vi "MIDI-Parser.vi"(8 "Error In":errorcluster, 11 "Consumer Data In":T3={"Queue_Consumer"=refnum, "Selected Consumer"=enum."Random", "Session Data"={"Tx-Data"=[], "Rx-Data"=[], "MIDI-Message log"=[{"Message Name"="", "Meta value"=0, "Datastring"="", "Datatype"=enum."No Data"}]}, "Timout-Time[ms]"=0, "To_GUI-Consumer"=refnum, "CPU(ms)"=0, "Console log"="", "MIDI Parse Data"={"MIDI-Bytes In"=[145, 60, 100], "MIDI Tag"=[], "MIDI Parsed Data"=[], "Iteration"=0, "Error?"=[], "Running States"=[], "Running Statusbyte"=0, "Running StatusString"="", "Third Byte Flag"=FALSE, "Current Byte"=0, "Sysex"="", "Expect Databyte"=FALSE}, "Session Inspection Data"={"Diff"=[], "Tx Byte"=[], "Rx Byte"=[], "Send Log"=[], "Parsed Data"={"Tx MIDI Tag"=[], "Tx MIDI Parsed Data"=[], "Tx Error"=[], "Tx Running States"=[], "Rx MIDI Tag"=[], "Rx MIDI Parsed Data"=[], "Rx Error"=[], "Rx Running States"=[], "Diff"=[]}}} {"MIDI Parse Data"."Current Byte" format="%.0x"; "MIDI Parse Data"."Running Statusbyte" format="%.0x"; "MIDI Parse Data"."MIDI-Bytes In" format="%.0x"}) -> (0 "Error Out":errorcluster, 3 "Consumer Data Out":T3={"Queue_Consumer"=refnum, "Selected Consumer"=enum."Random", "Session Data"={"Tx-Data"=[], "Rx-Data"=[], "MIDI-Message log"=[{"Message Name"="", "Meta value"=0, "Datastring"="", "Datatype"=enum."No Data"}]}, "Timout-Time[ms]"=0, "To_GUI-Consumer"=refnum, "CPU(ms)"=0, "Console log"="", "MIDI Parse Data"={"MIDI-Bytes In"=[145, 60, 100], "MIDI Tag"=[], "MIDI Parsed Data"=[], "Iteration"=0, "Error?"=[], "Running States"=[], "Running Statusbyte"=0, "Running StatusString"="", "Third Byte Flag"=FALSE, "Current Byte"=0, "Sysex"="", "Expect Databyte"=FALSE}, "Session Inspection Data"={"Diff"=[], "Tx Byte"=[], "Rx Byte"=[], "Send Log"=[], "Parsed Data"={"Tx MIDI Tag"=[], "Tx MIDI Parsed Data"=[], "Tx Error"=[], "Tx Running States"=[], "Rx MIDI Tag"=[], "Rx MIDI Parsed Data"=[], "Rx Error"=[], "Rx Running States"=[], "Diff"=[]}}} {"MIDI Parse Data"."Current Byte" format="%.0x"; "MIDI Parse Data"."Running Statusbyte" format="%.0x"; "MIDI Parse Data"."MIDI-Bytes In" format="%.0x"})   [LabVIEW 2019]
doc: "This parser constructs MIDI-messages from bytearray, by following the MIDI-spec."
uses:
  Controls/Parser-data.ctl
  Controls/Consumer_Data.ctl
  Common/Controls/Application_Message.ctl
  Common/Controls/Application_State.ctl
  Controls/Consumer_States.ctl
  Controls/Transfer_Data.ctl
  MIDI/Controls/MIDI-Message_Array.ctl
  MIDI/Controls/MIDI-Message_Cluster.ctl
  MIDI/Controls/Meta_Commands.ctl
  Controls/Consumer_Result.ctl
  Controls/Parsed_Data.ctl
  Controls/MIDI-States.ctl
panel:
  out "Control Tab":T1(tab)
  out "Console Out":string
  in  "MIDI Parse Data":T2={"MIDI-Bytes In"=[145, 60, 100], "MIDI Tag"=[], "MIDI Parsed Data"=[], "Iteration"=0, "Error?"=[], "Running States"=[], "Running Statusbyte"=0, "Running StatusString"="", "Third Byte Flag"=FALSE, "Current Byte"=0, "Sysex"="", "Expect Databyte"=FALSE} {"Current Byte" format="%.0x"; "Running Statusbyte" format="%.0x"; "MIDI-Bytes In" format="%.0x"}
  out "MIDI Tag":string[](array[string])
  out "MIDI Parsed Data":string[](array[string])
  out "Running States":string[](array[string])
  out "Error?":bool[](array[boolean])
  out "Error Message":string
  out "VI-filename":string
  out "Revision Number":u32
  out "VI Description":string
  out "Callers' Names":string[](array[string])
  out "Code Size":u32
  out "VI Type":T11(ring)
  out "Project name":string
  out "Project filepath":path
  out "VI filepath":path
  out "Project Description":string
  out "VI-Name":string
  in  "Stop":bool
  # "Common Errors:"
  # "0:"
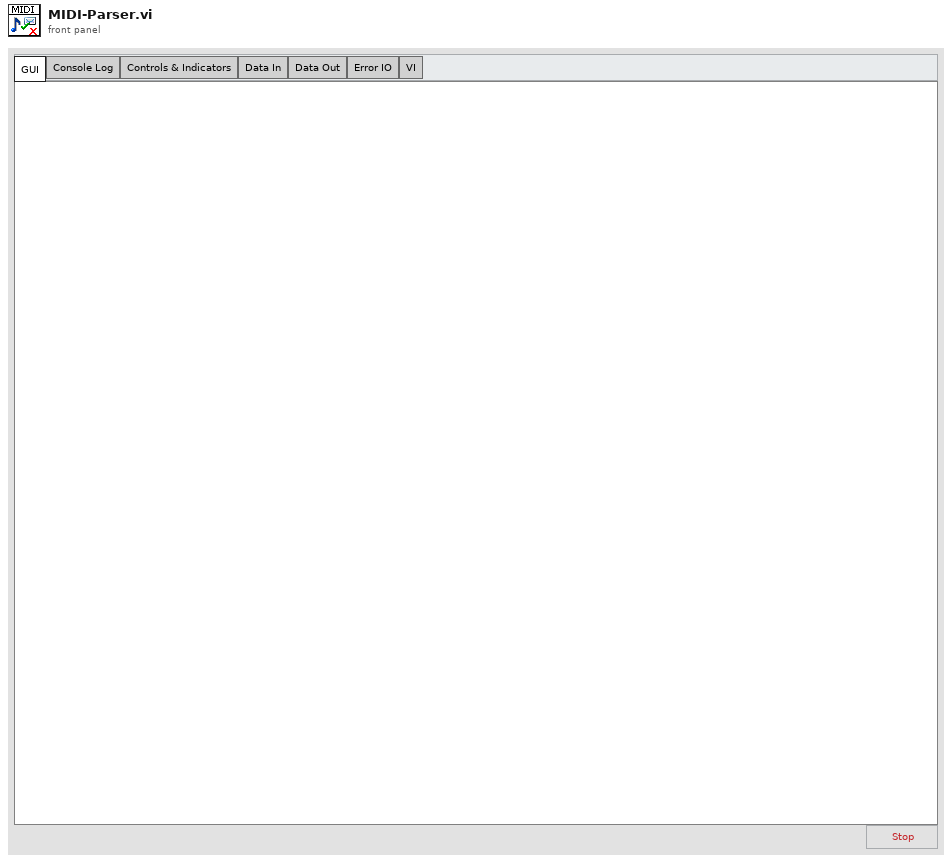
[diagram p1: front panel]
types:
  T1 = enum32{"GUI", "Console Log", "Controls & Indicators", "Data In", "Data Out", "Error IO", "VI"}
  T2 = typedef "Parser-data.ctl" = cluster{"MIDI-Bytes In":u8[], "MIDI Tag":string[], "MIDI Parsed Data":string[], "Iteration":i32, "Error?":bool[], "Running States":string[], "Running Statusbyte":u8, "Running StatusString":string, "Third Byte Flag":bool, "Current Byte":u8, "Sysex":string, "Expect Databyte":bool}
  T3 = typedef "Consumer_Data.ctl" = cluster{"Queue_Consumer":refnum<queue>, "Selected Consumer":T4, "Session Data":T5, "Timout-Time[ms]":i32, "To_GUI-Consumer":refnum<user-event>, "CPU(ms)":u32, "Console log":string, "MIDI Parse Data":T2, "Session Inspection Data":T9}
  T4 = typedef "Consumer_States.ctl" = enum16{"Random", "ECG", "Strech-Patch"}
  T5 = typedef "Transfer_Data.ctl" = cluster{"Tx-Data":i8[], "Rx-Data":i8[], "MIDI-Message log":T6}
  T6 = typedef "MIDI-Message_Array.ctl" = T7[]
  T7 = typedef "MIDI-Message_Cluster.ctl" = cluster{"Message Name":string, "Meta value":i32, "Datastring":string, "Datatype":T8}
  T8 = typedef "Meta_Commands.ctl" = enum16{"No Data", "Pause", "Loop", "Wait for Rx", "Delay", "Break", "MIDI"}
  T9 = typedef "Consumer_Result.ctl" = cluster{"Diff":bool[], "Tx Byte":string[], "Rx Byte":string[], "Send Log":string[], "Parsed Data":T10}
  T10 = typedef "Parsed_Data.ctl" = cluster{"Tx MIDI Tag":string[], "Tx MIDI Parsed Data":string[], "Tx Error":bool[], "Tx Running States":string[], "Rx MIDI Tag":string[], "Rx MIDI Parsed Data":string[], "Rx Error":bool[], "Rx Running States":string[], "Diff":bool[]}
  T11 = enum32{"invalid VI type", "Standard VI", "Control VI", "Global VI", "Polymorphic VI", "Configuration VI", "SubSystem", "Facade VI", "Method VI", "Statechart Diagram VI"}
  T12 = typedef "MIDI-States.ctl" = enum16{"Init Reset", "Dispatch Status", "SysEx"}
  T13 = typedef "LVRectTypeDef.ctl" = cluster{"Left":i16, "Top":i16, "Right":i16, "Bottom":i16}
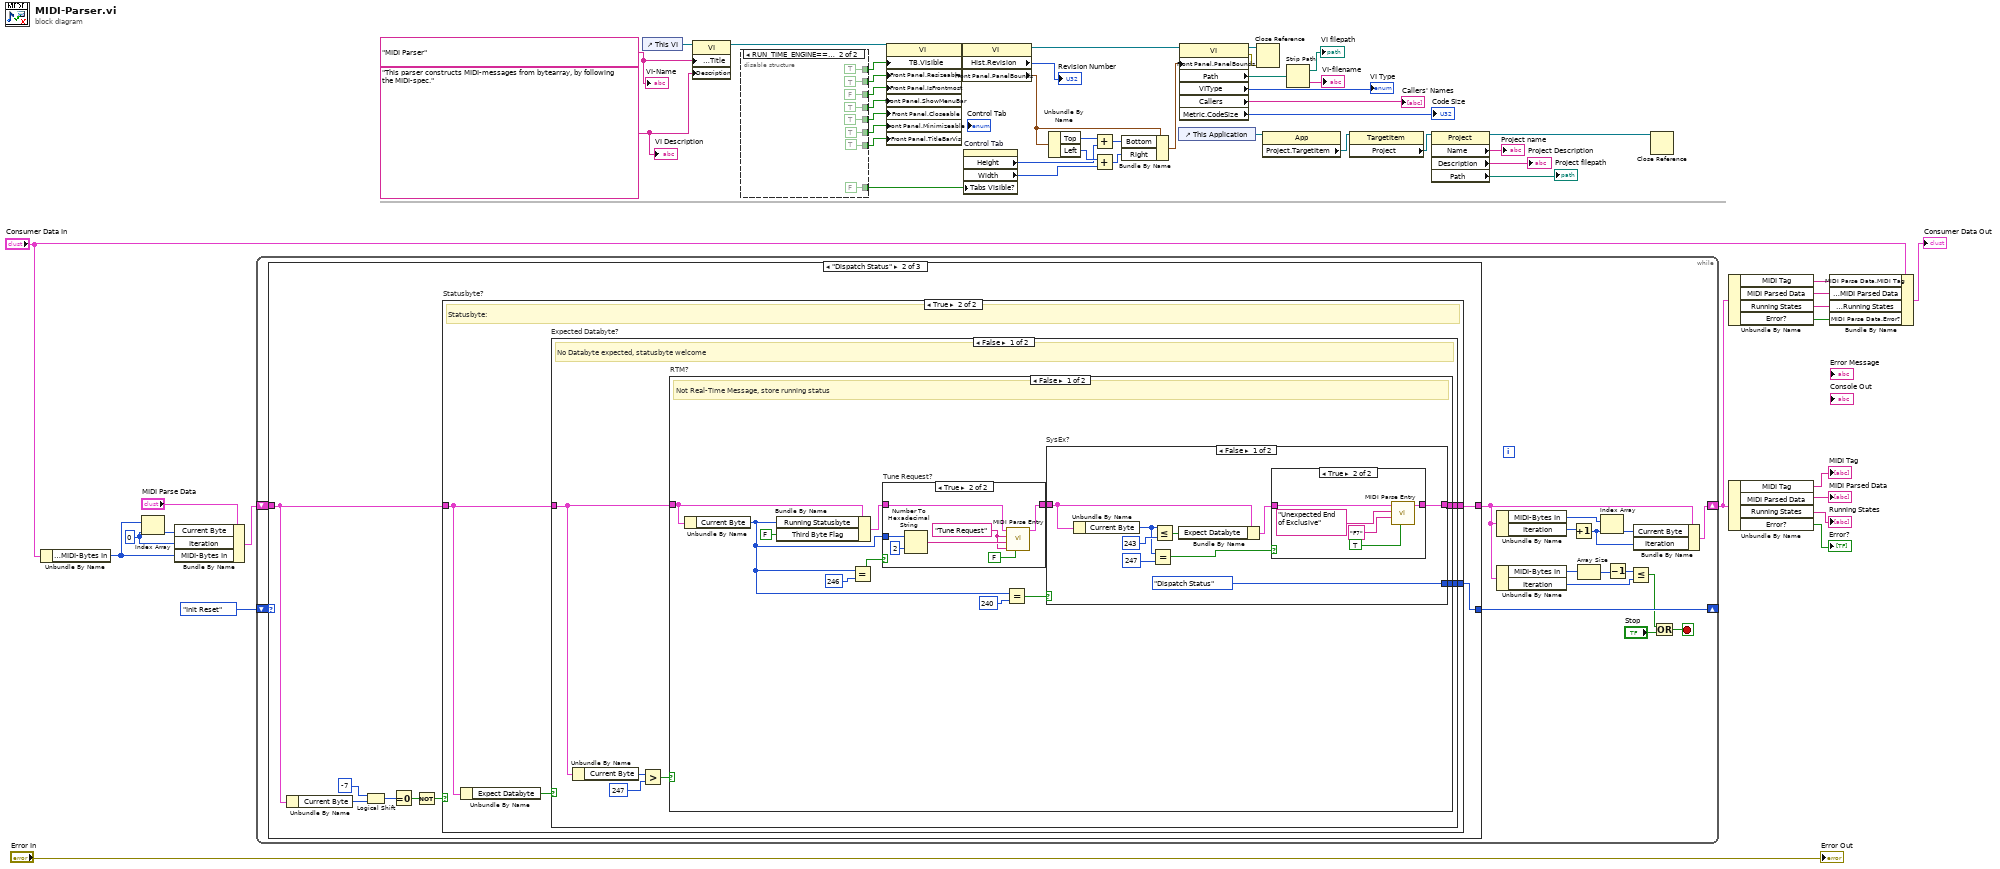
[diagram p0: block diagram]
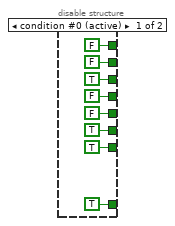
[diagram p2: hidden frame]
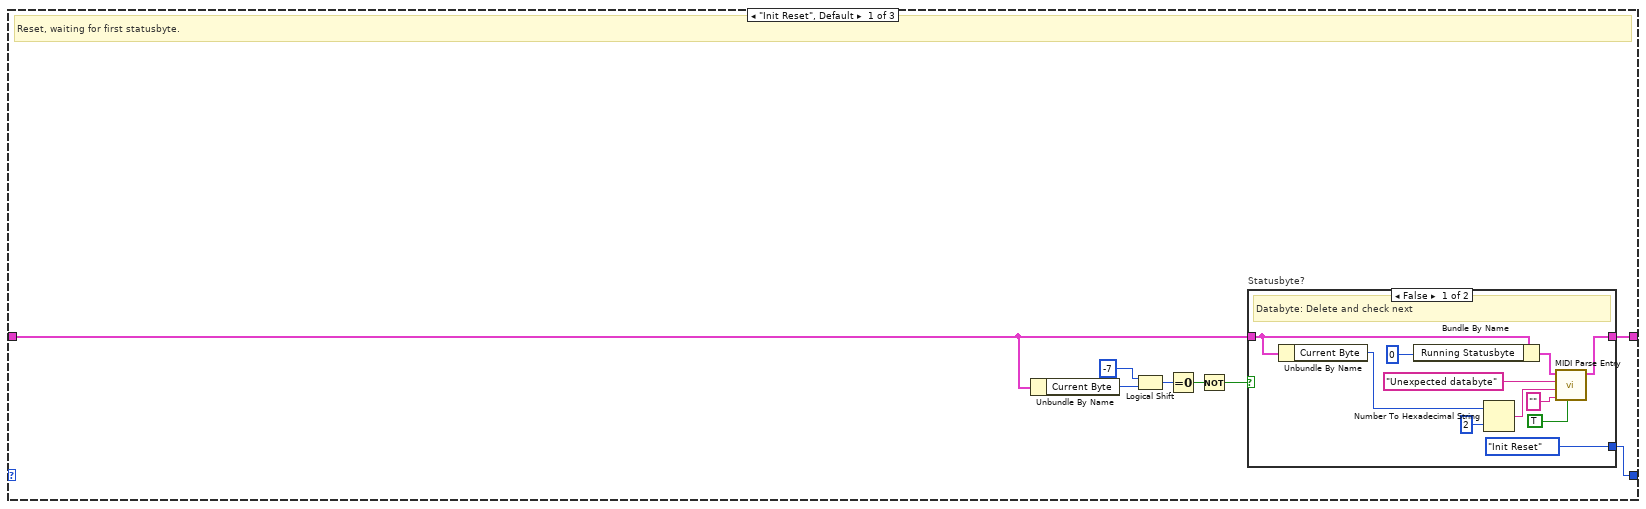
[diagram p3: hidden frame]
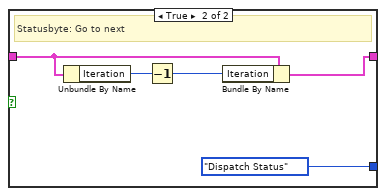
[diagram p4: hidden frame]
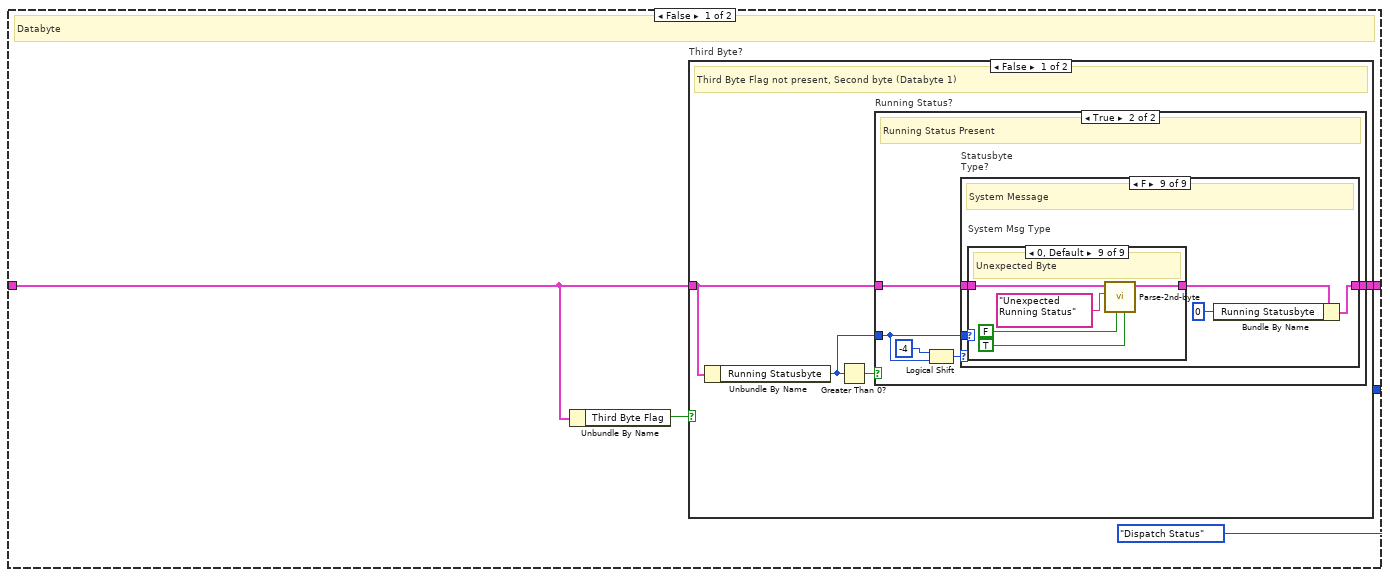
[diagram p5: hidden frame]
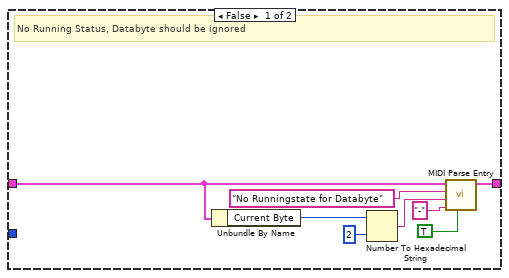
[diagram p6: hidden frame]
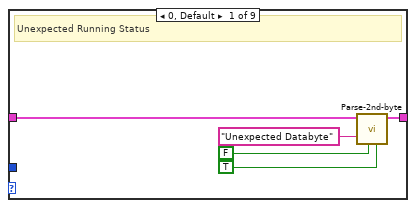
[diagram p7: hidden frame]
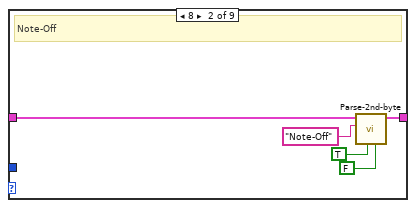
[diagram p8: hidden frame]
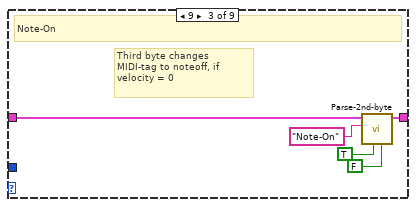
[diagram p9: hidden frame]
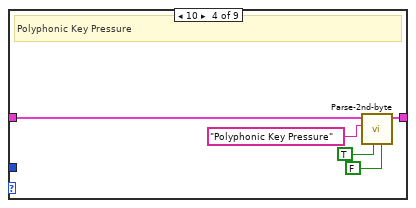
[diagram p10: hidden frame]
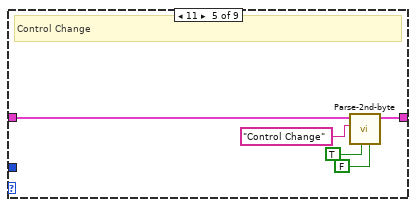
[diagram p11: hidden frame]
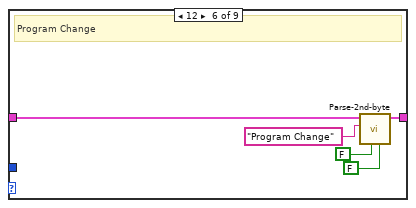
[diagram p12: hidden frame]
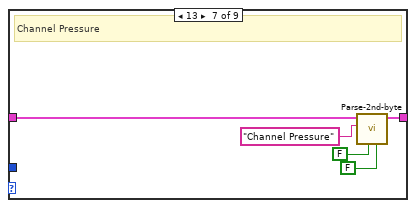
[diagram p13: hidden frame]
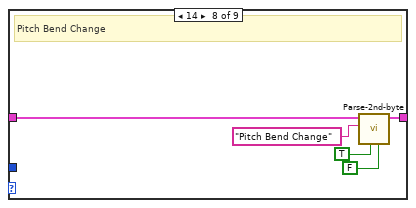
[diagram p14: hidden frame]
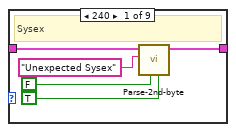
[diagram p15: hidden frame]
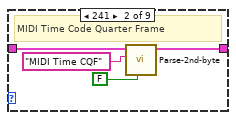
[diagram p16: hidden frame]
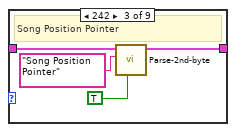
[diagram p17: hidden frame]
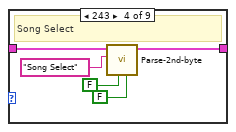
[diagram p18: hidden frame]
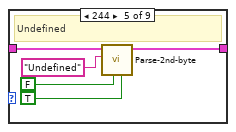
[diagram p19: hidden frame]
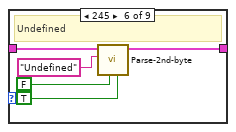
[diagram p20: hidden frame]
diagram:
  w42 = "MIDI Parser"
  w41 = "This parser constructs MIDI-messages from bytearray, by following the MIDI-spec."
  w52 = 0
  n1 = Unbundle By Name("Consumer Data In") -> ("MIDI Parse Data.MIDI-Bytes In"=w11:u8[])
  n2 = Index Array(array=w11, index=w52) -> (element=w51:u8)
  n3 = Bundle By Name(cluster="MIDI Parse Data", "Current Byte"=w51, "Iteration"=w52, "MIDI-Bytes In"=w11) -> (w56:T2)
  n4 = while {
    shift-right: [w67] -> w1
    shift-left: w56 -> [w72]
    shift-right: [w71] -> _
    shift-left: MIDI-States."Init Reset" -> [w73]
    stop <- w61 stop-if-true
    n5 = case shown="\"Dispatch Status\"" w73 {
      tunnel: w72 -> [w79 w101 w358]
      tunnel: [w78 w98 w355] -> w71
      tunnel: [w81 w100 w356] -> w65
      frame "Init Reset", Default {
        # "Reset, waiting for first statusbyte."
        n6 = Unbundle By Name(w79) -> ("Current Byte"=w80:u8)
        n7 = Logical Shift(y=i16 -7, x=w80) -> (x << y=w76:u8)
        n8 = Equal To 0?(x=w76) -> (x = 0?=w75:bool)
        n9 = Not(x=w75) -> (.not. x?=w74:bool)
        n10 = case "Statusbyte?" shown="False" w74 {
          tunnel: w79 -> [w86 w94]
          tunnel: [w84 w93] -> w81
          tunnel: [MIDI-States."Init Reset" MIDI-States."Dispatch Status"] -> w78
          frame False {
            # "Databyte: Delete and check next"
            n11 = Unbundle By Name(w86) -> ("Current Byte"=w82:u8)
            n12 = Bundle By Name(cluster=w86, "Running Statusbyte"=u8 0 ("Running Status")) -> (w85:T2)
            n13 = Number To Hexadecimal String(1:i16 2 ("width (-)"), 2:w82) -> (0:w87:string)
            n14 = call "MIDI Parse Entry.vi"("Error"=TRUE, "Running State"="", "Datastring"=w87, "MIDI Tag"="Unexpected databyte", "MIDI Parse Data in"=w85) -> ("MIDI Parse Data out"=w84:T2)  [unwired: 6 in]
          }
          frame True {
            # "Statusbyte: Go to next"
            n15 = Unbundle By Name(w94) -> ("Iteration"=w96:i32)
            n16 = Decrement(x=w96) -> (x-1=w95:i32)
            n17 = Bundle By Name(cluster=w94, "Iteration"=w95) -> (w93:T2)
          }
        }
      }
      frame "Dispatch Status" {
        n18 = Unbundle By Name(w101) -> ("Current Byte"=w99:u8)
        n19 = Logical Shift(y=i16 -7, x=w99) -> (x << y=w104:u8)
        n20 = Equal To 0?(x=w104) -> (x = 0?=w103:bool)
        n21 = Not(x=w103) -> (.not. x?=w102:bool)
        n22 = case "Statusbyte?" shown="True" w102 {
          tunnel: w101 -> [w108 w243]
          tunnel: [w107 w245] -> w100
          tunnel: [MIDI-States."Dispatch Status" w244] -> w98
          frame False {
            # "Databyte"
            n23 = Unbundle By Name(w108) -> ("Third Byte Flag"=w109:bool)
            n24 = case "Third Byte?" shown="False" w109 {
              tunnel: w108 -> [w112 w233]
              tunnel: [w110 w221] -> w107
              frame False {
                # "Third Byte Flag not present, Second byte (Databyte 1)"
                n25 = Unbundle By Name(w112) -> ("Running Statusbyte"=w111:u8)
                n26 = Greater Than 0?(x=w111) -> (x > 0?=w113:bool)
                n27 = case "Running Status?" shown="True" w113 {
                  tunnel: w112 -> [w115 w124]
                  tunnel: w111 -> [_ w123]
                  tunnel: [w114 w122] -> w110
                  frame False {
                    # "No Running Status, Databyte should be ignored"
                    n28 = Unbundle By Name(w115) -> ("Current Byte"=w116:u8)
                    n29 = Number To Hexadecimal String(1:i16 2 ("width (-)"), 2:w116) -> (0:w117:string)
                    n30 = call "MIDI Parse Entry.vi"("Error"=TRUE, "Running State"="-", "Datastring"=w117, "MIDI Tag"="No Runningstate for Databyte", "MIDI Parse Data in"=w115) -> ("MIDI Parse Data out"=w114:T2)  [unwired: 6 in]
                  }
                  frame True {
                    # "Running Status Present"
                    n31 = Logical Shift(y=i16 -4, x=w123) -> (x << y=w125:u8)
                    n32 = case "Statusbyte\nType?" shown="F" w125 {
                      tunnel: w124 -> [w129 w135 w140 w145 w150 w155 w160 w165 w170]
                      tunnel: w123 -> [_ _ _ _ _ _ _ _ w171]
                      tunnel: [w127 w134 w139 w146 w149 w154 w159 w164 w168] -> w122
                      frame 0, Default {
                        # "Unexpected Running Status"
                        n33 = call "Parse-2nd-byte.vi"("Error?"=TRUE, "Third Byte Flag"=FALSE, "Statustype"="Unexpected Databyte", "MIDI Parse Data in"=w129) -> ("MIDI Parse Data out"=w127:T2)  [unwired: 7 in]
                      }
                      frame 8 {
                        # "Note-Off"
                        n34 = call "Parse-2nd-byte.vi"("Error?"=FALSE, "Third Byte Flag"=TRUE, "Statustype"="Note-Off", "MIDI Parse Data in"=w135) -> ("MIDI Parse Data out"=w134:T2)  [unwired: 7 in]
                      }
                      frame 9 {
                        # "Third byte changes MIDI-tag to noteoff, if velocity = 0"
                        # "Note-On"
                        n35 = call "Parse-2nd-byte.vi"("Error?"=FALSE, "Third Byte Flag"=TRUE, "Statustype"="Note-On", "MIDI Parse Data in"=w140) -> ("MIDI Parse Data out"=w139:T2)  [unwired: 7 in]
                      }
                      frame 10 {
                        # "Polyphonic Key Pressure"
                        n36 = call "Parse-2nd-byte.vi"("Error?"=FALSE, "Third Byte Flag"=TRUE, "Statustype"="Polyphonic Key Pressure", "MIDI Parse Data in"=w145) -> ("MIDI Parse Data out"=w146:T2)  [unwired: 7 in]
                      }
                      frame 11 {
                        # "Control Change"
                        n37 = call "Parse-2nd-byte.vi"("Error?"=FALSE, "Third Byte Flag"=TRUE, "Statustype"="Control Change", "MIDI Parse Data in"=w150) -> ("MIDI Parse Data out"=w149:T2)  [unwired: 7 in]
                      }
                      frame 12 {
                        # "Program Change"
                        n38 = call "Parse-2nd-byte.vi"("Error?"=FALSE, "Third Byte Flag"=FALSE, "Statustype"="Program Change", "MIDI Parse Data in"=w155) -> ("MIDI Parse Data out"=w154:T2)  [unwired: 7 in]
                      }
                      frame 13 {
                        # "Channel Pressure"
                        n39 = call "Parse-2nd-byte.vi"("Error?"=FALSE, "Third Byte Flag"=FALSE, "Statustype"="Channel Pressure", "MIDI Parse Data in"=w160) -> ("MIDI Parse Data out"=w159:T2)  [unwired: 7 in]
                      }
                      frame 14 {
                        # "Pitch Bend Change"
                        n40 = call "Parse-2nd-byte.vi"("Error?"=FALSE, "Third Byte Flag"=TRUE, "Statustype"="Pitch Bend Change", "MIDI Parse Data in"=w165) -> ("MIDI Parse Data out"=w164:T2)  [unwired: 7 in]
                      }
                      frame 15 {
                        # "System Message"
                        n41 = case "System Msg Type" shown="0, Default" w171 {
                          tunnel: w170 -> [w174 w179 w182 w187 w191 w196 w202 w206 w211]
                          tunnel: [w173 w178 w181 w186 w190 w195 w201 w205 w210] -> w169
                          frame 240 {
                            # "Sysex"
                            n42 = call "Parse-2nd-byte.vi"("Error?"=TRUE, "Third Byte Flag"=FALSE, "Statustype"="Unexpected Sysex", "MIDI Parse Data in"=w174) -> ("MIDI Parse Data out"=w173:T2)  [unwired: 7 in]
                          }
                          frame 241 {
                            # "MIDI Time Code Quarter Frame"
                            n43 = call "Parse-2nd-byte.vi"("Third Byte Flag"=FALSE, "Statustype"="MIDI Time CQF", "MIDI Parse Data in"=w179) -> ("MIDI Parse Data out"=w178:T2)  [unwired: 8 in]
                          }
                          frame 242 {
                            # "Song Position Pointer"
                            n44 = call "Parse-2nd-byte.vi"("Third Byte Flag"=TRUE, "Statustype"="Song Position Pointer", "MIDI Parse Data in"=w182) -> ("MIDI Parse Data out"=w181:T2)  [unwired: 8 in]
                          }
                          frame 243 {
                            # "Song Select"
                            n45 = call "Parse-2nd-byte.vi"("Error?"=FALSE, "Third Byte Flag"=FALSE, "Statustype"="Song Select", "MIDI Parse Data in"=w187) -> ("MIDI Parse Data out"=w186:T2)  [unwired: 7 in]
                          }
                          frame 244 {
                            # "Undefined"
                            n46 = call "Parse-2nd-byte.vi"("Error?"=TRUE, "Third Byte Flag"=FALSE, "Statustype"="Undefined", "MIDI Parse Data in"=w191) -> ("MIDI Parse Data out"=w190:T2)  [unwired: 7 in]
                          }
                          frame 245 {
                            # "Undefined"
                            n47 = call "Parse-2nd-byte.vi"("Error?"=TRUE, "Third Byte Flag"=FALSE, "Statustype"="Undefined", "MIDI Parse Data in"=w196) -> ("MIDI Parse Data out"=w195:T2)  [unwired: 7 in]
                          }
                          frame 246 {
                            # "Tune Request"
                            n48 = call "Parse-2nd-byte.vi"("Error?"=TRUE, "Third Byte Flag"=FALSE, "Statustype"="Unexpected TQ", "MIDI Parse Data in"=w202) -> ("MIDI Parse Data out"=w201:T2)  [unwired: 7 in]
                          }
                          frame 247 {
                            # "End of Exclusive"
                            n49 = call "Parse-2nd-byte.vi"("Error?"=TRUE, "Third Byte Flag"=FALSE, "Statustype"="Unexpected End of Exclusive", "MIDI Parse Data in"=w206) -> ("MIDI Parse Data out"=w205:T2)  [unwired: 7 in]
                          }
                          frame 0, Default {
                            # "Unexpected Byte"
                            n50 = call "Parse-2nd-byte.vi"("Error?"=TRUE, "Third Byte Flag"=FALSE, "Statustype"="Unexpected Running Status", "MIDI Parse Data in"=w211) -> ("MIDI Parse Data out"=w210:T2)  [unwired: 7 in]
                          }
                        }
                        n51 = Bundle By Name(cluster=w169, "Running Statusbyte"=u8 0) -> (w168:T2)
                      }
                    }
                  }
                }
              }
              frame True {
                w215 = FALSE ("Third Byte Flag")
                # "Designate as Note off, if velocity is 0 on Note-on"
                # "Third byte"
                n52 = Unbundle By Name(w233) -> ("MIDI Parsed Data"=w235:string[], "Current Byte"=w216:u8, "MIDI Tag"=w225:string[], "Running Statusbyte"=w228:u8)
                n53 = Array Size(array=w235) -> (size(s)=w239:i32)
                n54 = Decrement(x=w239) -> (x-1=w238:i32)
                n55 = Logical Shift(y=i16 -4, x=w228) -> (x << y=w230:u8)
                n56 = Index Array(array=w235, index=w238) -> (element=w237:string)
                n57 = Number To Hexadecimal String(1:i16 2 ("width (-)"), 2:w216) -> (0:w240:string)
                n58 = Array Size(array=w225) -> (size(s)=w227:i32)
                n59 = Decrement(x=w227) -> (x-1=w226:i32)
                n60 = Array Size(array=w235) -> (size(s)=w234:i32)
                n61 = Replace Array Subset(array=w225, new element="Note-Off*" ("new element/subarray"), index=w226) -> (w224:string[])
                n62 = Concatenate Strings(w237, w240) -> (w236:string)
                n63 = Decrement(x=w234) -> (x-1=w220:i32)
                n64 = Equal?(x=w230, y=u8 9) -> (x = y?=w219:bool)
                n65 = Equal To 0?(x=w216) -> (x = 0?=w217:bool)
                n66 = Replace Array Subset(array=w235, new element=w236, index=w220) -> (w232:string[])
                n67 = And(x=w217, y=w219) -> (x .and. y?=w218:bool)
                n68 = Select(t=w224, s=w218, f=w225) -> (s? t:f=w222:string[])
                n69 = Bundle By Name(cluster=w233, "MIDI Parsed Data"=w232, "MIDI Tag"=w222, "Third Byte Flag"=w215, "Expect Databyte"=w215) -> (w221:T2)
              }
            }
          }
          frame True {
            # "Statusbyte:"
            n70 = Unbundle By Name(w243) -> ("Expect Databyte"=w242:bool)
            n71 = case "Expected Databyte?" shown="False" w242 {
              tunnel: w243 -> [w248 w312]
              tunnel: [w247 w313] -> w245
              tunnel: [w246 MIDI-States."Dispatch Status"] -> w244
              frame False {
                # "No Databyte expected, statusbyte welcome"
                n72 = Unbundle By Name(w248) -> ("Current Byte"=w251:u8)
                n73 = Greater?(x=w251, y=u8 247) -> (0:w249:bool)
                n74 = case "RTM?" shown="False" w249 {
                  tunnel: w248 -> [w262 w305]
                  tunnel: [w252 w291] -> w247
                  tunnel: [w254 w293] -> w246
                  frame False {
                    # "Not Real-Time Message, store running status"
                    n75 = Unbundle By Name(w262) -> ("Current Byte"=w256:u8)
                    n76 = Bundle By Name(cluster=w262, "Running Statusbyte"=w256, "Third Byte Flag"=FALSE) -> (w258:T2)
                    n77 = Equal?(x=w256, y=u8 246) -> (x = y?=w259:bool)
                    n78 = case "Tune Request?" shown="True" w259 {
                      tunnel: w256 -> [_ w289]
                      tunnel: w258 -> [w282 w285]
                      tunnel: [w282 w284] -> w253
                      frame False {
                      }
                      frame True {
                        w286 = "Tune Request" ("MIDI Tag")
                        n79 = Number To Hexadecimal String(1:i16 2 ("width (-)"), 2:w289) -> (0:w287:string)
                        n80 = call "MIDI Parse Entry.vi"("Error"=FALSE, "Running State"=w286, "Datastring"=w287, "MIDI Tag"=w286, "MIDI Parse Data in"=w285) -> ("MIDI Parse Data out"=w284:T2)  [unwired: 6 in]
                      }
                    }
                    n81 = Equal?(x=w256, y=u8 240) -> (x = y?=w255:bool)
                    n82 = case "SysEx?" shown="False" w255 {
                      tunnel: [MIDI-States."Dispatch Status" ("f") MIDI-States."SysEx"] -> w254
                      tunnel: w253 -> [w269 w280]
                      tunnel: [w263 w279] -> w252
                      frame False {
                        n83 = Unbundle By Name(w269) -> ("Current Byte"=w267:u8)
                        n84 = Equal?(x=w267, y=u8 247) -> (x = y?=w264:bool)
                        n85 = Less Or Equal?(x=w267, y=u8 243) -> (x <= y?=w270:bool)
                        n86 = Bundle By Name(cluster=w269, "Expect Databyte"=w270) -> (w265:T2)
                        n87 = case shown="True" w264 {
                          tunnel: w265 -> [w272 w276]
                          tunnel: [w272 w277] -> w263
                          frame False {
                          }
                          frame True {
                            n88 = call "MIDI Parse Entry.vi"("Error"=TRUE, "Datastring"="F7", "MIDI Tag"="Unexpected End of Exclusive", "MIDI Parse Data in"=w276) -> ("MIDI Parse Data out"=w277:T2)  [unwired: 7 in]
                          }
                        }
                      }
                      frame True {
                        n89 = Bundle By Name(cluster=w280, "Expect Databyte"=TRUE) -> (w279:T2)
                      }
                    }
                  }
                  frame True {
                    # "System Real-Time Message, no running Status. If Reset, do so..."
                    n90 = Unbundle By Name(w305) -> ("Current Byte"=w306:u8, "Running StatusString"=w304:string)
                    n91 = Subtract(x=w306, y=u8 248) -> (x-y=w299:u8)
                    n92 = Number To Hexadecimal String(1:i16 2 ("width (-)"), 2:w306) -> (0:w307:string)
                    n93 = Index Array(array=string[] ["Timing Clock", "Undefined", "Start", "Continue", "Stop", "Undefined", "Active Sensing", "Reset"], index=w299) -> (element=w295:string)
                    n94 = Concatenate Strings("RTM " ("string"), w295) -> (w294:string)
                    n95 = Equal?(x=w306, y=u8 255) -> (x = y?=w302:bool)
                    n96 = Select(t=MIDI-States."Init Reset", s=w302, f=MIDI-States."Dispatch Status") -> (s? t:f=w293:T12)
                    n97 = call "MIDI Parse Entry.vi"("Error"=FALSE, "Running State"=w304, "Datastring"=w307, "MIDI Tag"=w294, "MIDI Parse Data in"=w305) -> ("MIDI Parse Data out"=w292:T2)  [unwired: 6 in]
                    n98 = Bundle By Name(cluster=w292, "Expect Databyte"=FALSE) -> (w291:T2)
                  }
                }
              }
              frame True {
                w316 = FALSE ("Third Byte Flag")
                n99 = Unbundle By Name(w312) -> ("Third Byte Flag"=w311:bool)
                n100 = case "Databytes Expected" shown="True" w311 {
                  tunnel: w312 -> [w326 w347]
                  tunnel: [w327 w346] -> w310
                  frame False {
                    # "1 Databyte expected"
                    n101 = Unbundle By Name(w326) -> ("MIDI Parsed Data"=w331:string[], "Running Statusbyte"=w334:u8, "MIDI Tag"=w329:string[], "Error?"=w323:bool[], "Running States"=w320:string[])
                    n102 = Number To Hexadecimal String(1:i16 2 ("width (-)"), 2:w334) -> (0:w332:string)
                    n103 = Insert Into Array(array=w320, new element="-" ("new element/subarray")) -> (w319:string[])  [unwired: 1 in]
                    n104 = Concatenate Strings(w332, "xx" ("string")) -> (w330:string)
                    n105 = Insert Into Array(array=w329, new element="Expected Databyte" ("MIDI Tag")) -> (w324:string[])  [unwired: 1 in]
                    n106 = Insert Into Array(array=w331, new element=w330) -> (w325:string[])  [unwired: 1 in]
                    n107 = Insert Into Array(array=w323, new element=TRUE ("new element/subarray")) -> (w321:bool[])  [unwired: 1 in]
                    n108 = Bundle By Name(cluster=w326, "MIDI Parsed Data"=w325, "MIDI Tag"=w324, "Error?"=w321, "Running States"=w319) -> (w327:T2)
                  }
                  frame True {
                    # "2 Databytes expected"
                    n109 = Unbundle By Name(w347) -> ("MIDI Parsed Data"=w354:string[], "MIDI Tag"=w353:string[], "Error?"=w349:bool[], "Running States"=w338:string[])
                    n110 = Array Size(array=w354) -> (size(s)=w351:i32)
                    n111 = Subtract(x=w351, y=1) -> (x-y=w336:i32)
                    n112 = Index Array(array=w354, index=w336) -> (element=w343:string)
                    n113 = Replace Array Subset(array=w353, new element="Expected Databyte" ("MIDI Tag"), index=w336) -> (w344:string[])
                    n114 = Replace Array Subset(array=w349, new element=TRUE ("new element/subarray"), index=w336) -> (w340:bool[])
                    n115 = Replace Array Subset(array=w338, new element="-" ("new element/subarray"), index=w336) -> (w339:string[])
                    n116 = Concatenate Strings(w343, "xx" ("string")) -> (w342:string)
                    n117 = Replace Array Subset(array=w354, new element=w342, index=w336) -> (w345:string[])
                    n118 = Bundle By Name(cluster=w347, "MIDI Parsed Data"=w345, "MIDI Tag"=w344, "Error?"=w340, "Running States"=w339) -> (w346:T2)
                  }
                }
                n119 = Unbundle By Name(w310) -> ("Iteration"=w315:i32)
                n120 = Decrement(x=w315) -> (x-1=w314:i32)
                n121 = Bundle By Name(cluster=w310, "Iteration"=w314, "Third Byte Flag"=w316, "Expect Databyte"=w316) -> (w313:T2)
              }
            }
          }
        }
      }
      frame "SysEx" {
        n122 = Unbundle By Name(w358) -> ("Current Byte"=w357:u8)
        n123 = Logical Shift(y=i16 -7, x=w357) -> (x << y=w361:u8)
        n124 = Equal To 0?(x=w361) -> (x = 0?=w360:bool)
        n125 = Not(x=w360) -> (.not. x?=w359:bool)
        n126 = case "Statusbyte?" shown="False" w359 {
          tunnel: w358 -> [w365 w374]
          tunnel: [w364 w375] -> w356
          tunnel: w357 -> [_ w378]
          tunnel: [MIDI-States."SysEx" MIDI-States."Dispatch Status"] -> w355
          frame False {
            # "Concatenate untill end of exclusive."
            # "Databyte, Continue storing/concatenating"
            n127 = Unbundle By Name(w365) -> ("Sysex"=w370:string, "Current Byte"=w369:u8)
            n128 = Number To Hexadecimal String(1:i16 2 ("width (-)"), 2:w369) -> (0:w367:string)
            n129 = Concatenate Strings(w370, w367) -> (w366:string)
            n130 = Bundle By Name(cluster=w365, "Sysex"=w366) -> (w364:T2)
          }
          frame True {
            # "Statusbyte, check if \"End of Exclusive\""
            n131 = Unbundle By Name(w374) -> ("Running Statusbyte"=w381:u8, "Sysex"=w382:string)
            n132 = Number To Hexadecimal String(1:i16 2 ("width (-)"), 2:w381) -> (0:w379:string)
            n133 = Concatenate Strings(w379, w382) -> (w373:string)
            n134 = Bundle By Name(cluster=w374, "Sysex"=w373) -> (w372:T2)
            n135 = Equal?(x=w378, y=u8 247) -> (x = y?=w376:bool)
            n136 = case "End of Exclusive?" shown="True" w376 {
              tunnel: w372 -> [w393 w416]
              tunnel: [w385 w408] -> w375
              frame True {
                # "Store and continue"
                n137 = Unbundle By Name(w393) -> ("MIDI Parsed Data"=w399:string[], "Sysex"=w403:string, "Current Byte"=w402:u8, "MIDI Tag"=w397:string[], "Error?"=w395:bool[], "Running States"=w388:string[])
                n138 = Number To Hexadecimal String(1:i16 2 ("width (-)"), 2:w402) -> (0:w400:string)
                n139 = Concatenate Strings(w403, w400) -> (w398:string)
                n140 = Insert Into Array(array=w399, new element=w398) -> (w392:string[])  [unwired: 1 in]
                n141 = Insert Into Array(array=w397, new element="SysEx" ("new element/subarray")) -> (w391:string[])  [unwired: 1 in]
                n142 = Insert Into Array(array=w395, new element=FALSE ("new element/subarray")) -> (w390:bool[])  [unwired: 1 in]
                n143 = Insert Into Array(array=w388, new element="-" ("new element/subarray")) -> (w387:string[])  [unwired: 1 in]
                n144 = Bundle By Name(cluster=w393, "MIDI Parsed Data"=w392, "MIDI Tag"=w391, "Error?"=w390, "Running Statusbyte"=u8 0, "Running States"=w387, "Sysex"="", "Expect Databyte"=FALSE) -> (w385:T2)
              }
              frame False {
                # "Store and continue"
                n145 = Unbundle By Name(w416) -> ("Iteration"=w406:i32, "MIDI Parsed Data"=w421:string[], "Sysex"=w422:string, "MIDI Tag"=w420:string[], "Error?"=w418:bool[], "Running States"=w411:string[])
                n146 = Insert Into Array(array=w421, new element=w422) -> (w415:string[])  [unwired: 1 in]
                n147 = Insert Into Array(array=w420, new element="Aborted SysEx" ("new element/subarray")) -> (w414:string[])  [unwired: 1 in]
                n148 = Insert Into Array(array=w418, new element=TRUE ("new element/subarray")) -> (w413:bool[])  [unwired: 1 in]
                n149 = Insert Into Array(array=w411, new element="-" ("new element/subarray")) -> (w410:string[])  [unwired: 1 in]
                n150 = Decrement(x=w406) -> (x-1=w405:i32)
                n151 = Bundle By Name(cluster=w416, "Iteration"=w405, "MIDI Parsed Data"=w415, "MIDI Tag"=w414, "Error?"=w413, "Running Statusbyte"=u8 0, "Running States"=w410, "Sysex"="", "Expect Databyte"=FALSE) -> (w408:T2)
              }
            }
          }
        }
      }
    }
    n152 = Unbundle By Name(w65) -> ("MIDI-Bytes In"=w69:u8[], "Iteration"=w70:i32)
    n153 = Unbundle By Name(w65) -> ("MIDI-Bytes In"=w62:u8[], "Iteration"=w64:i32)
    n154 = Increment(x=w70) -> (x+1=w66:i32)
    n155 = Array Size(array=w62) -> (size(s)=w63:i32)
    n156 = Index Array(array=w69, index=w66) -> (element=w68:u8)
    n157 = Decrement(x=w63) -> (x-1=w58:i32)
    n158 = Less Or Equal?(x=w58, y=w64) -> (x <= y?=w59:bool)
    n159 = Bundle By Name(cluster=w65, "Current Byte"=w68, "Iteration"=w66) -> (w67:T2)
    n160 = Or(x=w59, y="Stop") -> (x .or. y?=w61:bool)
  }
  n161 = control-ref of="This VI"() -> (w43:refnum<vi>)
  n162 = property class="VI"(reference=w43, "Front Panel.Title"=w42, "Description"=w41) -> (reference out=w40:refnum<vi>)  [unwired: 1 in, 1 out]
  n163 = disable-structure "Exe vs Sim" shown="RUN_TIME_ENGINE==True" {
    disable-tunnel: [FALSE ("Tool Bar:Visible") TRUE ("Tool Bar:Visible")] -> w44
    disable-tunnel: [FALSE ("Front Panel Window:Resizable") TRUE ("Front Panel Window:Resizable")] -> w45
    disable-tunnel: [TRUE ("Front Panel Window:Is Frontmost") FALSE ("Front Panel Window:Is Frontmost")] -> w46
    disable-tunnel: [FALSE ("Front Panel Window:Show Menu Bar") TRUE ("Front Panel Window:Show Menu Bar")] -> w47
    disable-tunnel: [FALSE ("Front Panel Window:Closeable") TRUE ("Front Panel Window:Closeable")] -> w48
    disable-tunnel: [TRUE ("Front Panel Window:Title Bar Visible") TRUE ("Front Panel Window:Title Bar Visible")] -> w49
    disable-tunnel: [TRUE ("Front Panel Window:Minimizable") TRUE ("Front Panel Window:Minimizable")] -> w50
    disable-tunnel: [TRUE FALSE] -> w39
    frame condition #0 (active) {
    }
    frame condition #1 {
    }
  }
  n164 = property class="VI"(reference=w40, "TB.Visible"=w44, "Front Panel.Resizeable"=w45, "Front Panel.IsFrontmost"=w46, "Front Panel.ShowMenuBar"=w47, "Front Panel.Closeable"=w48, "Front Panel.Minimizeable"=w50, "Front Panel.TitleBarVis"=w49) -> (reference out=w38:refnum<vi>, error out=w37:errorcluster)  [unwired: 1 in]
  n165 = property class="VI"(reference=w38, error in=w37) -> (reference out=w28:refnum<vi>, "Hist.Revision"=→"Revision Number":u32, "Front Panel.PanelBounds"=w30:T13)  [unwired: 1 out]
  n166 = property on="Control Tab" class="TabCtl (strict)"("Tabs Visible?"=w39) -> ("Height"=w32:u32, "Width"=w31:u32)  [unwired: 2 in, 2 out]
  n167 = Unbundle By Name(w30) -> ("Top"=w36:i16, "Left"=w33:i16)
  n168 = Add(x=w36, y=w32) -> (x+y=w35:u32)
  n169 = Add(x=w33, y=w31) -> (x+y=w34:u32)
  n170 = Bundle By Name(cluster=w30, "Bottom"=w35, "Right"=w34) -> (w27:T13)
  n171 = control-ref of="This Application"() -> (w18:refnum<vi>)
  n172 = property on="Window size" class="VI"(reference=w28, "Front Panel.PanelBounds"=w27) -> (reference out=w26:refnum<vi>, error out=w25:errorcluster, "Path"=w24:path, "VIType"=→"VI Type":T11, "Callers"=→"Callers' Names":string[], "Metric.CodeSize"=→"Code Size":u32)  [unwired: 1 in]
  n173 = Close Reference(reference=w26, error in (no error)=w25) -> ()  [unwired: 1 out]
  n174 = property class="App"(reference=w18) -> ("Project.TargetItem"=w16:refnum<vi>)  [unwired: 1 in, 2 out]
  n175 = Strip Path(path=w24) -> (stripped path=→"VI filepath":path, name=→"VI-filename":string)
  n176 = property class="TargetItem"(reference=w16) -> ("Project"=w17:refnum<vi>)  [unwired: 1 in, 2 out]
  n177 = property class="Project"(reference=w17) -> (reference out=w12:refnum<vi>, "Name"=→"Project name":string, "Description"=→"Project Description":string, "Path"=→"Project filepath":path)  [unwired: 1 in, 1 out]
  n178 = Close Reference(reference=w12) -> ()  [unwired: 1 in, 1 out]
  n179 = Unbundle By Name(w1) -> ("MIDI Tag"=w5:string[], "MIDI Parsed Data"=w4:string[], "Running States"=w3:string[], "Error?"=w2:bool[])
  n180 = Unbundle By Name(w1) -> ("MIDI Tag"=→"MIDI Tag":string[], "MIDI Parsed Data"=→"MIDI Parsed Data":string[], "Running States"=→"Running States":string[], "Error?"=→"Error?":bool[])
  n181 = Bundle By Name(cluster="Consumer Data In", "MIDI Parse Data.MIDI Tag"=w5, "MIDI Parse Data.MIDI Parsed Data"=w4, "MIDI Parse Data.Running States"=w3, "MIDI Parse Data.Error?"=w2) -> (→"Consumer Data Out":T3)
  "VI Description" <- w41
  "VI-Name" <- w42
  "Error Out" <- "Error In"
